vi "Get Joystick.vi"(8 "error in (no error)":errorcluster, 11 "XBoxController-P in":refnum<class "XBoxController-P.lvclass">) -> (0 "error out":errorcluster, 3 "XBoxController-P out":refnum<class "XBoxController-P.lvclass">)   [LabVIEW 2013, in "XBoxController-P.lvclass"]
uses:
  XBoxController-P.lvclass
  Logical Systems/XBoxController/XBoxController.lvclass
  XBoxController-P.lvclass/XBoxController-P.ctl
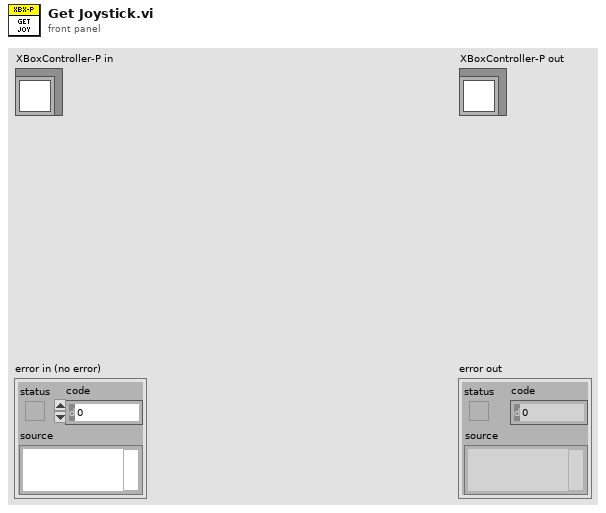
[diagram p1: front panel]
types:
  T1 = typedef "WPI_JoystickDevRef.ctl" = cluster{"Device":T2}
  T2 = typedef "WPI_JoystickDeviceEnum.ctl" = enum16{"USB 1", "USB 2", "USB 3", "USB 4", "Kinect 1", "Kinect 2"}
  T3 = typedef "WPI_JoystickButtonState.ctl" = cluster{"Button 1":bool, "Button 2":bool, "Button 3":bool, "Button 4":bool, "Button 5":bool, "Button 6":bool, "Button 7":bool, "Button 8":bool, "Button 9":bool, "Button 10":bool, "Button 11":bool, "Button 12":bool}
  T4 = cluster{"axis 1 (x)":dbl, "axis 2 (y)":dbl, "axis 3 (throttle)":dbl, "axis 4":dbl, "axis 5":dbl, "axis 6":dbl}
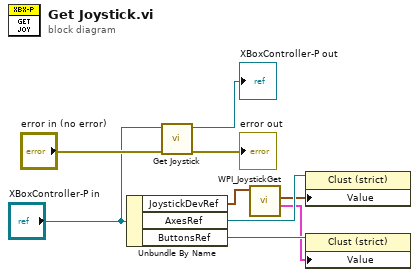
[diagram p0: block diagram]
diagram:
  n1 = Unbundle By Name("XBoxController-P in") -> ("JoystickDevRef"=w5:T1, "AxesRef"=w4:refnum<vi>, "ButtonsRef"=w2:refnum<vi>)
  n2 = call-parent "Get Joystick.vi"("error in (no error)"="error in (no error)", "XBoxController in"="XBoxController-P in") -> ("error out"=→"error out":errorcluster, "XBoxController out"=→"XBoxController-P out":refnum<class "XBoxController-P.lvclass">)  [unwired: 8 in]
  n3 = call <vilib>:"WPI_JoystickGet.vi"("JoystickDevRef"=w5) -> ("Buttons"=w1:T3, "Axes"=w3:T4)  [unwired: 4 in, 1 out]
  n4 = property class="Clust (strict)"(reference=w4, "Value"=w3) -> ()  [unwired: 1 in, 2 out]
  n5 = property class="Clust (strict)"(reference=w2, "Value"=w1) -> ()  [unwired: 1 in, 2 out]
